vi "Update GUI - Append String.vi"(4 "Append to bottom":bool=TRUE, 6 "Lines to keep":u8=30, 8 "error in (no error)":errorcluster, 9 "String":string, 10 "GUI Item Name":string, 11 "Father of all uServices in":refnum<class "Father of all uServices.lvclass">) -> (0 "error out":errorcluster, 3 "Father of all uServices out":refnum<class "Father of all uServices.lvclass">)   [LabVIEW 2026, in "TALOS.lvlib" / "Father of all uServices.lvlib" / "Father of all uServices.lvclass"]
doc: "Use this VI to append a string to a string indicator: between the existing string and the added one a linefeed will be added. With the parameter Line to keep you can specify how many lines do you want to keep in the indicator (default: 42)."
uses:
  Father of all uServices.lvclass
  Father of all uServices.lvclass/Father of all uServices.ctl
  Ancestor/Ancestor/Ancestor.lvclass/Ancestor.ctl
  Support VIs/Substitute Error.vi
  Support VIs/Generate Error.vi
  FGV/Error Memory/Get Error Description.vi
  Support VIs/Get PC name.vi
  Ancestor/Ancestor/Read ID.vi
  Support VIs/Get Class Name.vi
  <vilib>/Utility/error.llb/Clear Errors.vi
  FGV/Error Memory/Error Memory Core.vi
  <vilib>/AdvancedString/Delimited String to 1D String Array.vi
  <vilib>/AdvancedString/Delimited String to 1D String Array (string).vi
  Support VIs/Circus Root Path.vi
  FGV/Error Memory/Error Crt Lvl checker.vi
  FGV/Error Memory/Error Memory Core.vi/40c8088d-b597-4017-91af-faa98e00292e.vi
  FGV/Error Memory/Error Memory Core.vi/d4a3ab98-063c-4e44-b43d-fbdcfe6c2be2.vi
  Support VIs/Global Memory.vi
  <vilib>/Utility/LVClass/Get LV Class Name.vi
  Support VIs/Is in Packed Library.vi
  Support VIs/TALOS Root path.vi
  Support VIs/Read CSV worksheet.vi
  Support VIs/Global Constants.vi
  <vilib>/Utility/error.llb/General Error Handler.vi
  Support VIs/Error Log.vi
  Ancestor/Ancestor/Ancestor.lvclass
  <vilib>/Comparison/Equal/Equal Functor/Equal Functor.lvclass
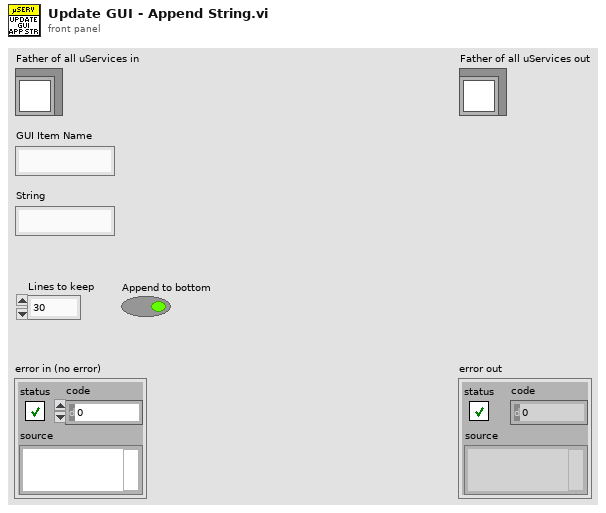
[diagram p1: front panel]
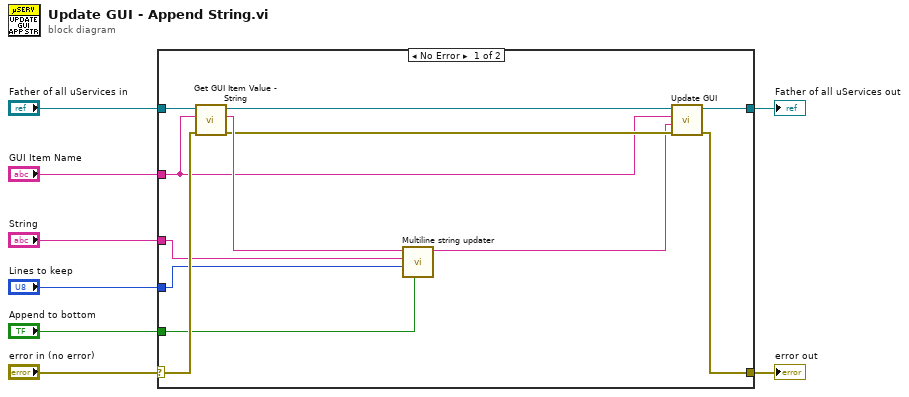
[diagram p0: block diagram]
diagram:
  n1 = case shown="No Error" "error in (no error)" {
    selector: "error in (no error)" -> [w20 w22]
    tunnel: [w10 w22] -> w7
    tunnel: [w14 w21] -> w5
    tunnel: "Father of all uServices in" -> [w19 w21]
    tunnel: "GUI Item Name" -> [w12 _]
    tunnel: "String" -> [w16 _]
    tunnel: "Lines to keep" -> [w17 _]
    tunnel: "Append to bottom" -> [w9 _]
    frame No Error {
      n2 = call "Get GUI Item Value - String.vi"("error in (no error)"=w20, "FP Item Name"=w12, "uService Template in"=w19) -> ("error out"=w13:errorcluster, "Value"=w18:string, "uService Template out"=w15:refnum<class "Father of all uServices.lvclass">)  [unwired: 6 in]
      n3 = call "Multiline string updater.vi"("Append to bottom"=w9, "Lines to keep"=w17, "String to add"=w16, "Multiline string in"=w18) -> ("Multiline string out"=w11:string)  [unwired: 7 in]
      n4 = call "Update GUI.vi"("error in (no error)"=w13, "Data"=w11, "GUI Item Name"=w12, "uService Template in"=w15) -> ("error out"=w10:errorcluster, "uService Template out"=w14:refnum<class "Father of all uServices.lvclass">)  [unwired: 6 in]
    }
    frame Error {
    }
  }
  "error out" <- w7
  "Father of all uServices out" <- w5
